vi "Expression Operand Throw.vi"(0 "operand":string, 2 "Exception Operand.lvclass":refnum<class "Exception Operand.lvclass">, 11 "error in (no error)":errorcluster) -> (4 "Exception Operand out":refnum<class "Exception Operand.lvclass">, 15 "error out":errorcluster)   [LabVIEW 2015, in "Exception Operand.lvclass"]
uses:
  Exception Operand.lvclass
  <userlib>/LV Exceptions v1/Exception/Exception.lvclass/Exception.ctl
  <vilib>/Utility/error.llb/Trim Whitespace.vi
  <userlib>/LV Exceptions v1/Exception/Exception.lvclass
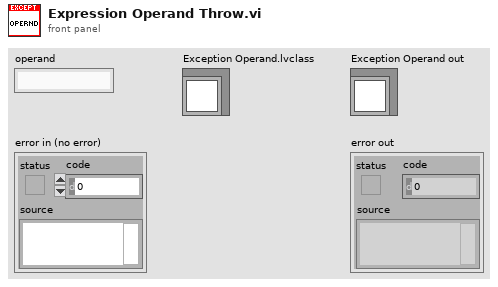
[diagram p1: front panel]
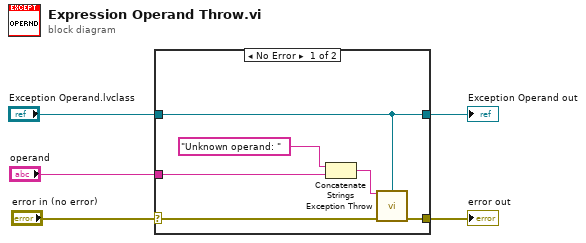
[diagram p0: block diagram]
diagram:
  n1 = case shown="No Error" "error in (no error)" {
    selector: "error in (no error)" -> [w11 w13]
    tunnel: [w10 w13] -> w4
    tunnel: [w9 w12] -> w3
    tunnel: "Exception Operand.lvclass" -> [w9 w12]
    tunnel: "operand" -> [w6 _]
    frame No Error {
      n2 = Concatenate Strings("Unknown operand: " ("message"), w6) -> (w7:string)
      n3 = call <userlib>:"Exception Throw.vi"("message"=w7, "Exception in"=w9, "error in (no error)"=w11) -> ("error out"=w10:errorcluster)  [unwired: 12 in]
    }
    frame Error {
    }
  }
  "error out" <- w4
  "Exception Operand out" <- w3
